vi "Set Ring Exposure Times.vi"(8 "error in (no error)":errorcluster, 10 "times":sgl, 11 "numTimes":i32) -> (0 "error out":errorcluster, 2 "times out":sgl, 3 "function return":u32)   [LabVIEW 2014, in "atmcd32d.lvlib"]
doc: "unsigned int WINAPI SetRingExposureTimes(int numTimes, float * times);"
uses:
  atmcd32d.lvlib
  atmcd32d.dll
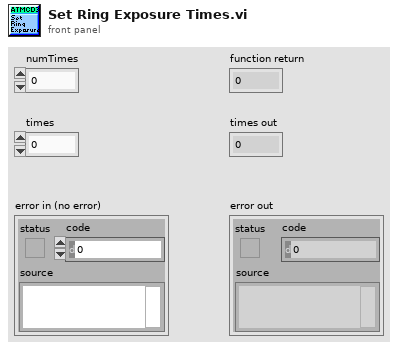
[diagram p1: front panel]
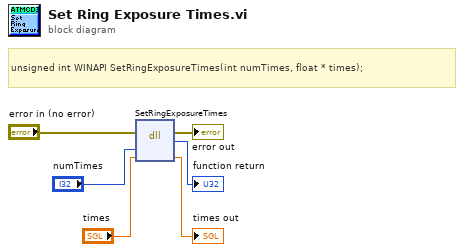
[diagram p0: block diagram]
diagram:
  # "unsigned int WINAPI SetRingExposureTimes(int numTimes, float * times);"
  n1 = dll-call lib="C:/Users/Bakir/Documents/Lambda2-Testing/lib/Andorlib/atmcd32d.*" fn="SetRingExposureTimes"(error in="error in (no error)", "numTimes"="numTimes", "times"="times") -> (error out=→"error out":errorcluster, →"function return":u32, "times"=→"times out":sgl)  [unwired: 3 in, 1 out]
